vi "Swerve Teleop.vi"(0 "X":dbl, 1 "Rot. Point X":dbl, 3 "Rot. Point Y":dbl, 5 "Y":dbl, 7 "Z":dbl, 11 "Error In":errorcluster, 12 "Robot Centric?":bool=TRUE, 13 "Autonomous?":bool) -> (4 "Front Left Output":dbl, 6 "Front Right Output":dbl, 8 "Back Left Output":dbl, 10 "Back Right Output":dbl, 15 "Error Out":errorcluster)   [LabVIEW 2016]
uses:
  <vilib>/Rock Robotics/Network Tables/NT Read Number.vi
  Robot Global Data.vi
  <vilib>/Rock Robotics/Network Tables/NT Write Numeric Array.vi
panel:
  in  "Robot Length":dbl=33.5
  in  "Robot Width":dbl=28.5
  # "Swerve Drive Teleoperated Control\nFRC Team 34"
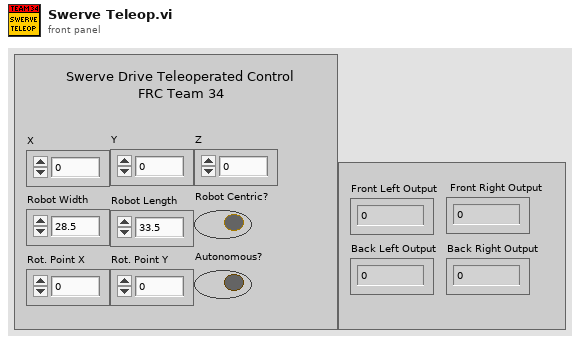
[diagram p1: front panel]
types:
  T1 = enum16{"Front Left", "Front Right", "Back Left", "Back Right"}
  T2 = cluster{"Yaw":dbl, "Roll":dbl, "Pitch":dbl, "Heading":dbl, "Fused Heading":dbl}
  T3 = typedef "WPI_MotorControlDeviceRef.ctl" = cluster{"DeviceStatus":errorcluster, "Type":T4, "PWM":cluster{"PWM Channel":T5, "DeadBand":T6}, "CAN":cluster{"Device Number":u8, "SetOutput VI Ref":variant, "GetOutput VI Ref":variant, "Enable VI Ref":variant, "Disable VI Ref":variant, "Data":variant}, "Invert":bool}
  T4 = typedef "WPI_MotorControlType.ctl" = enum16{"PWM", "CAN"}
  T5 = typedef "FPGA_DIOPWMChannel.ctl" = enum8{"PWM 0", "PWM 1", "PWM 2", "PWM 3", "PWM 4", "PWM 5", "PWM 6", "PWM 7", "PWM 8", "PWM 9", "PWM MXP 0", "PWM MXP 1", "PWM MXP 2", "PWM MXP 3", "PWM MXP 4", "PWM MXP 5", "PWM MXP 6", "PWM MXP 7", "PWM MXP 8", "PWM MXP 9", "Invalid"}
  T6 = typedef "WPI_PWMDeadband.ctl" = cluster{"Name":string, "maxPositivePwm":i32, "minPositivePwm":i32, "centerPwm":i32, "maxNegativePwm":i32, "minNegativePwm":i32, "angularRange":u16}
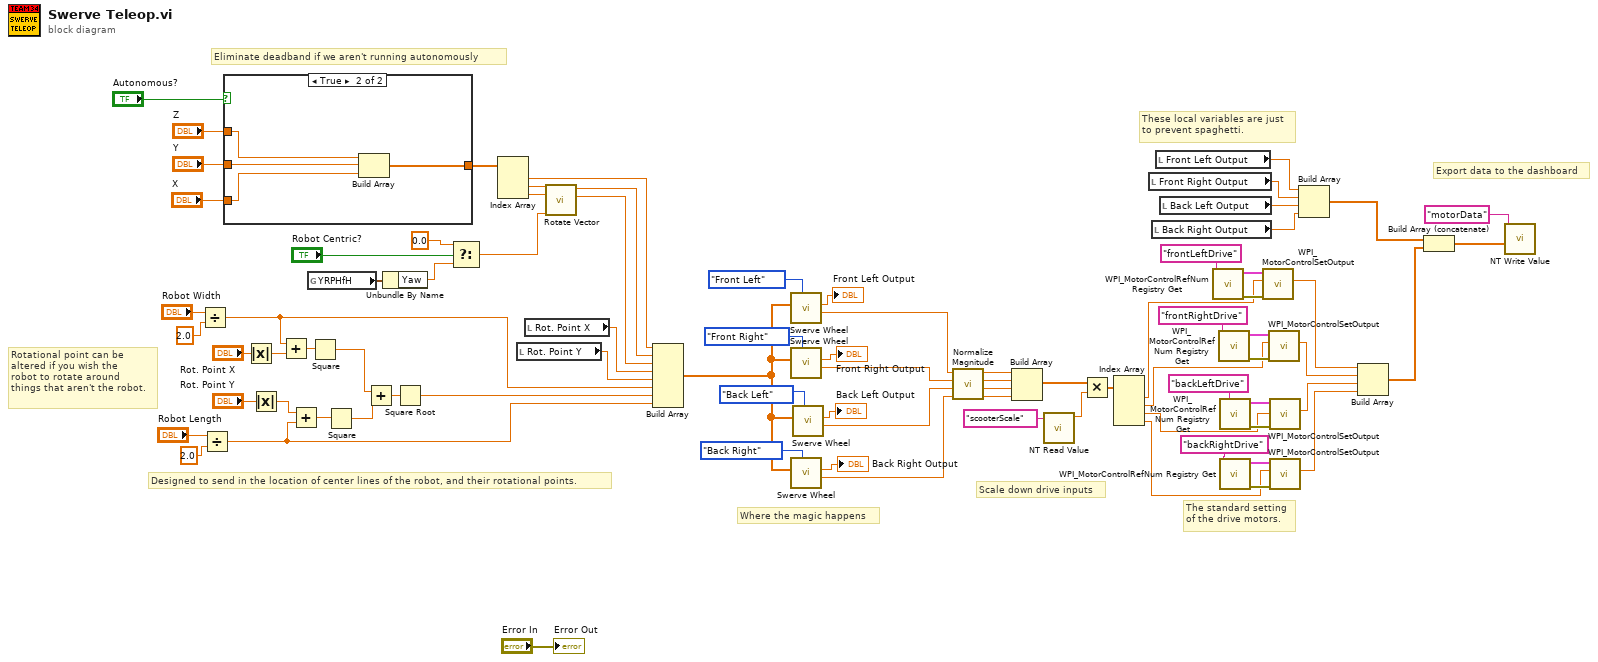
[diagram p0: block diagram]
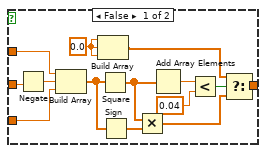
[diagram p2: hidden frame]
diagram:
  # "Rotational point can be \naltered if you wish the \nrobot to rotate around \nthings that aren't the robot."
  # "Scale down drive inputs"
  # "Eliminate deadband if we aren't running autonomously"
  # "These local variables are just \nto prevent spaghetti."
  # "Export data to the dashboard"
  # "Where the magic happens"
  # "The standard setting\nof the drive motors."
  # "Designed to send in the location of center lines of the robot, and their rotational points."
  n1 = Divide(x="Robot Width", y=2.0) -> (x/y=w54:dbl)
  n2 = Divide(x="Robot Length", y=2.0) -> (x/y=w52:dbl)
  n3 = case shown="True" "Autonomous?" {
    tunnel: "Y" -> [w87 w100]
    tunnel: [w86 w98] -> w82
    tunnel: "Z" -> [w85 w101]
    tunnel: "X" -> [w84 w99]
    frame False {
      w93 = 0.0 ("element")
      n4 = Negate(x=w87) -> (-x=w89:dbl)
      n5 = Build Array(w85, w89, w84) -> (w92:dbl[])
      n6 = Build Array(w93, w93, w93) -> (w94:dbl[])
      n7 = Square(x=w92) -> (x^2=w90:dbl[])
      n8 = Sign(1:w92) -> (0:w91:dbl[])
      n9 = Multiply(x=w90, y=w91) -> (x*y=w88:dbl[])
      n10 = Add Array Elements(numeric array=w90) -> (sum=w97:dbl)
      n11 = Less?(x=w97, y=0.04 ("x")) -> (x < y?=w95:bool)
      n12 = Select(t=w94, s=w95, f=w88) -> (s? t:f=w86:dbl[])
    }
    frame True {
      n13 = Build Array(w101, w100, w99) -> (w98:dbl[])
    }
  }
  n14 = Absolute Value(x="Rot. Point X") -> (abs(x)=w66:dbl)
  n15 = Absolute Value(x="Rot. Point Y") -> (abs(x)=w63:dbl)
  n16 = Add(x=w54, y=w66) -> (x+y=w65:dbl)
  n17 = Add(x=w63, y=w52) -> (x+y=w64:dbl)
  n18 = global read "Robot Global Data.vi" "YRPHfH"() -> (w80:T2)
  n19 = Square(x=w65) -> (x^2=w61:dbl)
  n20 = Square(x=w64) -> (x^2=w62:dbl)
  n21 = Add(x=w61, y=w62) -> (x+y=w60:dbl)
  n22 = Unbundle By Name(w80) -> ("Yaw"=w79:dbl)
  n23 = Square Root(x=w60) -> (sqrt(x)=w53:dbl)
  n24 = Select(t=0.0, s="Robot Centric?", f=w79) -> (s? t:f=w73:dbl)
  n25 = Index Array(array=w82) -> (element #1=w59:dbl, element #2=w75:dbl, element #3=w74:dbl)  [unwired: 3 in]
  n26 = local read "Rot. Point Y"() -> (w55:dbl)
  n27 = local read "Rot. Point X"() -> (w56:dbl)
  n28 = call "Rotate Vector.vi"("Angle"=w73, "X"=w74, "Y"=w75) -> ("X'"=w57:dbl, "Y'"=w58:dbl)  [unwired: 7 in]
  n29 = Build Array(w59, w58, w57, w56, w55, w54, w53, w52) -> (w51:dbl[])
  n30 = call "Swerve Wheel.vi"("Wheel"=T1."Front Left", "Inputs"=w51) -> ("Speed"=w46:dbl, "Motor Output"=→"Front Left Output":dbl)  [unwired: 8 in]
  n31 = call "Swerve Wheel.vi"("Wheel"=T1."Front Right", "Inputs"=w51) -> ("Speed"=w45:dbl, "Motor Output"=→"Front Right Output":dbl)  [unwired: 8 in]
  n32 = call "Swerve Wheel.vi"("Wheel"=T1."Back Right", "Inputs"=w51) -> ("Speed"=w43:dbl, "Motor Output"=→"Back Right Output":dbl)  [unwired: 8 in]
  n33 = call "Swerve Wheel.vi"("Wheel"=T1."Back Left", "Inputs"=w51) -> ("Speed"=w44:dbl, "Motor Output"=→"Back Left Output":dbl)  [unwired: 8 in]
  n34 = call "Normalize Magnitude.vi"("D"=w43, "C"=w44, "B"=w45, "A"=w46) -> ("D'"=w19:dbl, "C'"=w20:dbl, "B'"=w21:dbl, "A'"=w22:dbl)  [unwired: 4 in]
  n35 = Build Array(w22, w21, w20, w19) -> (w18:dbl[])
  n36 = call-poly <vilib>:"NT Read Value.vi"("Name"="scooterScale") -> ("Numeric"=w16:dbl)  [unwired: 9 in, 1 out]
  n37 = Multiply(x=w18, y=w16) -> (x*y=w15:dbl[])
  n38 = Index Array(array=w15) -> (element #1=w14:dbl, element #2=w13:dbl, element #3=w12:dbl, element #4=w11:dbl)  [unwired: 4 in]
  n39 = local read "Front Right Output"() -> (w4:dbl)
  n40 = local read "Back Right Output"() -> (w2:dbl)
  n41 = local read "Front Left Output"() -> (w5:dbl)
  n42 = local read "Back Left Output"() -> (w3:dbl)
  n43 = call <vilib>:"WPI_MotorControlRefNum Registry Get.vi"("refnum name"="frontLeftDrive") -> ("error out"=w41:errorcluster, "MotorControlDevRef"=w40:T3)  [unwired: 9 in]
  n44 = call <vilib>:"WPI_MotorControlRefNum Registry Get.vi"("refnum name"="frontRightDrive") -> ("error out"=w36:errorcluster, "MotorControlDevRef"=w39:T3)  [unwired: 9 in]
  n45 = call <vilib>:"WPI_MotorControlRefNum Registry Get.vi"("refnum name"="backLeftDrive") -> ("error out"=w35:errorcluster, "MotorControlDevRef"=w37:T3)  [unwired: 9 in]
  n46 = call <vilib>:"WPI_MotorControlRefNum Registry Get.vi"("refnum name"="backRightDrive") -> ("error out"=w33:errorcluster, "MotorControlDevRef"=w32:T3)  [unwired: 9 in]
  n47 = call <vilib>:"WPI_MotorControlSetOutput.vi"("error in (no error)"=w41, "Output"=w14, "MotorControlDevRef"=w40) -> ("Motor Output"=w30:dbl)  [unwired: 6 in, 2 out]
  n48 = call <vilib>:"WPI_MotorControlSetOutput.vi"("error in (no error)"=w36, "Output"=w13, "MotorControlDevRef"=w39) -> ("Motor Output"=w29:dbl)  [unwired: 6 in, 2 out]
  n49 = call <vilib>:"WPI_MotorControlSetOutput.vi"("error in (no error)"=w35, "Output"=w12, "MotorControlDevRef"=w37) -> ("Motor Output"=w28:dbl)  [unwired: 6 in, 2 out]
  n50 = call <vilib>:"WPI_MotorControlSetOutput.vi"("error in (no error)"=w33, "Output"=w11, "MotorControlDevRef"=w32) -> ("Motor Output"=w27:dbl)  [unwired: 6 in, 2 out]
  n51 = Build Array(w5, w4, w3, w2) -> (w25:dbl[])
  n52 = Build Array(w30, w29, w28, w27) -> (w26:dbl[])
  n53 = Build Array (concatenate)(w25, w26) -> (w24:dbl[])
  n54 = call-poly <vilib>:"NT Write Value.vi"("Numeric Array"=w24, "Name"="motorData") -> ()  [unwired: 9 in, 1 out]
  "Error Out" <- "Error In"
